vi "String Subset.vi"(3 "Offset past End":i32=-1, 4 "Start offset":i32, 5 "JSON":string) -> (1 "substring":string)   [LabVIEW 2015, in "JSONtext.lvlib"]
uses:
  JSONtext.lvlib
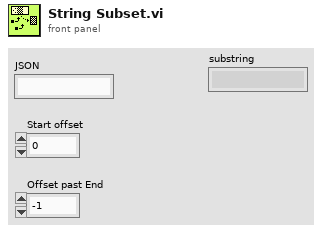
[diagram p1: front panel]
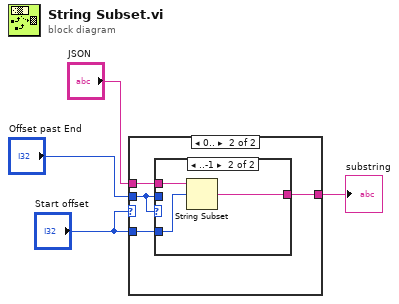
[diagram p0: block diagram]
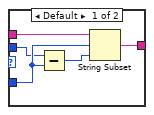
[diagram p3: hidden frame]
diagram:
  n1 = case shown="0.." "Start offset" {
    tunnel: "Start offset" -> [_ w6]
    tunnel: "Offset past End" -> [_ w5]
    tunnel: "JSON" -> [_ w8]
    tunnel: [_ w7] -> w2
    frame ..-1 {
    }
    frame 0.. {
      n2 = case shown="..-1" w5 {
        tunnel: w6 -> [w12 w16]
        tunnel: w5 -> [w11 _]
        tunnel: w8 -> [w10 w15]
        tunnel: [w9 w14] -> w7
        frame Default {
          n3 = Subtract(x=w11, y=w12) -> (x-y=w13:i32)
          n4 = String Subset(string=w10, offset (0)=w12, length (rest)=w13) -> (substring=w9:string)
        }
        frame ..-1 {
          n5 = String Subset(string=w15, offset (0)=w16) -> (substring=w14:string)  [unwired: 1 in]
        }
      }
    }
  }
  "substring" <- w2
